vi "Write Key Value I32.vi"(7 "Section Name":string, 8 "error in (no error)":errorcluster, 9 "Value":i32, 10 "Key Name":string, 11 "ODBC-Interface in":refnum<class "ODBC-Interface.lvclass">) -> (0 "error out":errorcluster, 2 "found":bool, 3 "ODBC-Interface out":refnum<class "ODBC-Interface.lvclass">)   [LabVIEW 2012, in "DB-Configuration.lvlib" / "ODBC-Interface.lvclass"]
doc: "Write I32 key value."
uses:
  ODBC-Interface.lvclass
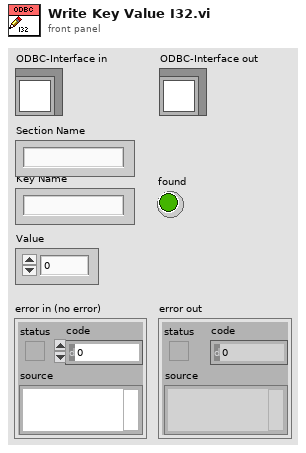
[diagram p1: front panel]
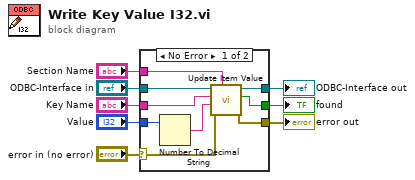
[diagram p0: block diagram]
diagram:
  n1 = case shown="No Error" "error in (no error)" {
    selector: "error in (no error)" -> [w10 w18]
    tunnel: "Section Name" -> [w17 _]
    tunnel: "ODBC-Interface in" -> [w16 w19]
    tunnel: [w15 w19] -> w3
    tunnel: "Key Name" -> [w14 _]
    tunnel: "Value" -> [w9 _]
    tunnel: [w12 w18] -> w1
    tunnel: [w11 _] -> w2
    frame No Error {
      n2 = Number To Decimal String(number=w9) -> (decimal integer string=w13:string)  [unwired: 1 in]
      n3 = call-dynamic "Update Item Value.vi"("Section Name"=w17, "error in (no error)"=w10, "Value"=w13, "Key Name"=w14, "ODBC-Interface in"=w16) -> ("error out"=w12:errorcluster, "found"=w11:bool, "ODBC-Interface out"=w15:refnum<class "ODBC-Interface.lvclass">)  [unwired: 4 in]
    }
    frame Error {
    }
  }
  "error out" <- w1
  "ODBC-Interface out" <- w3
  "found" <- w2
